vi "Configure Process Display and Static Message.vi"(0 "VISA resource name":refnum<visa-resource-name>, 1 "Unit Address (1)":i16=1, 5 "Input 1 Only (0: Input 1)":u16(ring) items=["Input 1", "Alternating"], 7 "Alternating Display Times (0.0; 0.0; 0.0)":dbl[](array[numeric]) format="%.2f", 9 "Static Messages (no strings)":string[](array[string]), 11 "error in (no error)":errorcluster {"code" format="%.0x"}) -> (4 "VISA resource name out":refnum<visa-resource-name>, 15 "error out":errorcluster {"code" format="%.0x"})   [LabVIEW 2010]
doc: "This VI configures process display and static messages."
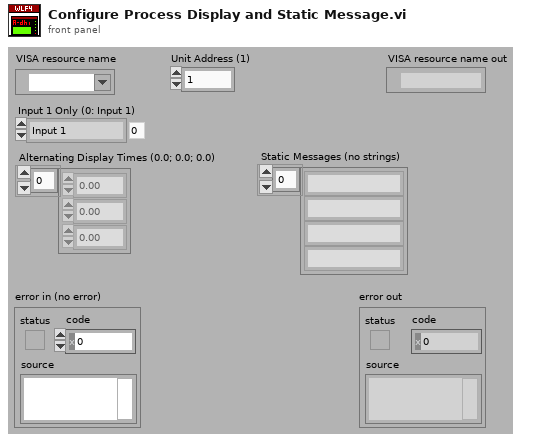
[diagram p1: front panel]
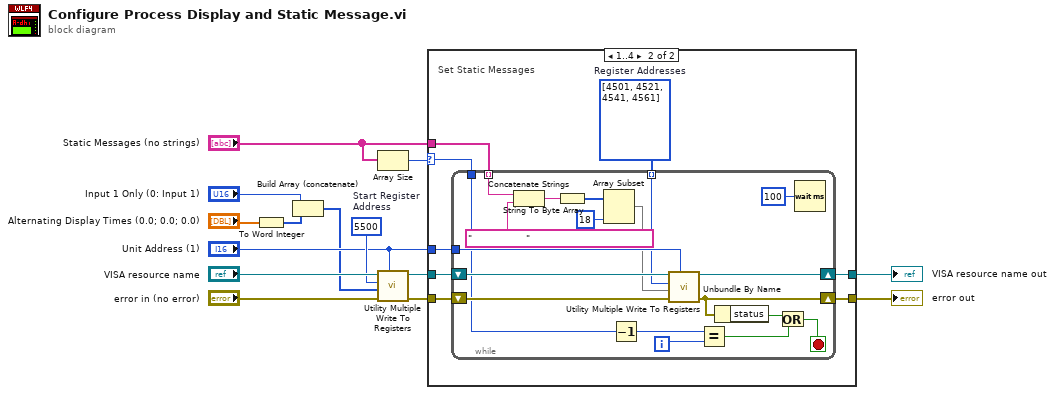
[diagram p0: block diagram]
diagram:
  w12 = u16 5500  # Start Register Address
  n1 = To Word Integer(number="Alternating Display Times (0.0; 0.0; 0.0)") -> (16bit integer=w4:i16[])
  n2 = Build Array (concatenate)("Input 1 Only (0: Input 1)", w4) -> (w3:u16[])
  n3 = Array Size(array="Static Messages (no strings)") -> (size(s)=w2:i32)
  n4 = call "Utility Multiple Write To Registers.vi"("Unit Address (1)"="Unit Address (1)", "error in (no error)"="error in (no error)", "Array Of Data"=w3, "Register Address (0)"=w12, "VISA resource name"="VISA resource name") -> ("error out"=w11:errorcluster, "VISA resource name out"=w10:refnum<visa-resource-name>)  [unwired: 5 in]
  n5 = case shown="1..4" w2 {
    selector: w2 -> [_ w17]
    tunnel: w11 -> [w15 w24]
    tunnel: w10 -> [w16 w23]
    tunnel: [w16 w22] -> w9
    tunnel: [w15 w21] -> w8
    tunnel: "Unit Address (1)" -> [_ w20]
    tunnel: "Static Messages (no strings)" -> [_ w18]
    frame 0, Default {
      # "No Static Message"
    }
    frame 1..4 {
      w19 = i32[] [4501, 4521, 4541, 4561]  # Register Addresses
      # "Set Static Messages"
      n6 = while {
        tunnel: w20 -> [w38]
        shift-right: [w36] -> w22
        shift-left: w23 -> [w37]
        shift-right: [w35] -> w21
        shift-left: w24 -> [w34]
        tunnel: w19 -> [w33] mode=indexing
        tunnel: w18 -> [w28] mode=indexing
        tunnel: w17 -> [w25]
        i -> [w40]
        stop <- w42 stop-if-true
        n7 = Concatenate Strings(w28, "                  " ("string")) -> (w31:string)
        n8 = String To Byte Array(string=w31) -> (unsigned byte array=w30:u8[])
        n9 = Array Subset(array=w30, length=18) -> (w27:u8[])  [unwired: 1 in]
        n10 = Decrement(x=w25) -> (x-1=w26:i32)
        n11 = call "Utility Multiple Write To Registers.vi"("Unit Address (1)"=w38, "error in (no error)"=w34, "Array Of Data"=w27, "Register Address (0)"=w33, "VISA resource name"=w37) -> ("error out"=w35:errorcluster, "VISA resource name out"=w36:refnum<visa-resource-name>)  [unwired: 5 in]
        n12 = Equal?(x=w26, y=w40) -> (x = y?=w39:bool)
        n13 = Unbundle By Name(w35) -> ("status"=w41:bool)
        n14 = Or(x=w41, y=w39) -> (x .or. y?=w42:bool)
        n15 = Wait (ms)(milliseconds to wait=u32 100) -> ()  [unwired: 1 out]
      }
    }
  }
  "error out" <- w8
  "VISA resource name out" <- w9
